vi "Convert PID Gains (PD).vi"(0 "proportional":sgl, 1 "gains pattern (Parallel)":T4=1 items=["Academic", "Parallel", "Series"], 2 "filter coefficient (NaN)":sgl=nan, 3 "filter coefficient unit (Alpha)":T1 items=["Alpha", "N", "Cutoff Frequency", "Time Constant"], 7 "derivative":sgl, 9 "sampling time":sgl min=0, 11 "error in (no error)":errorcluster, 12 "proportional unit (Gain (K))":T3 items=["Gain (K)", "Band (PB)"], 14 "derivative unit (s)":T2=1 items=["Hz", "s", "min"]) -> (4 "gains":T5 {"proportional gain" step=0.125}, 15 "error out":errorcluster)   [LabVIEW 2020]
doc: "Converts PID gains in the Academic, Parallel, or Series form to the normalized Parallel form that the PID VI expects."
uses:
  <vilib>/rvi/Analysis/control/PID/Typedef/niFpgaPID_PDGains.ctl
  <vilib>/rvi/Analysis/host/Private/PID Gains Pattern.ctl
  <vilib>/rvi/Analysis/host/Private/PID Proportional Unit.ctl
  <vilib>/rvi/Analysis/host/Private/PID Integral Derivative Unit.ctl
  <vilib>/rvi/Analysis/host/Private/PID Filter Coefficient Unit.ctl
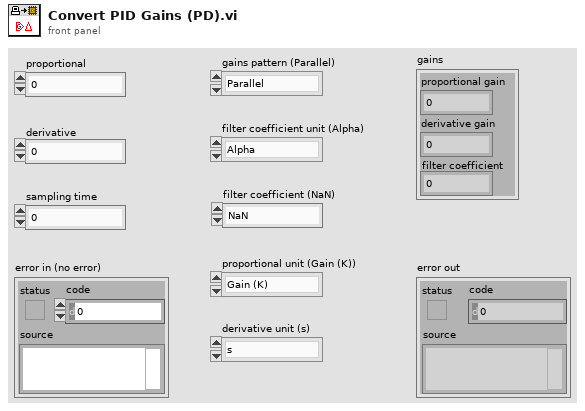
[diagram p1: front panel]
types:
  T1 = typedef "PID Filter Coefficient Unit.ctl" = u8
  T2 = typedef "PID Integral Derivative Unit.ctl" = u8
  T3 = typedef "PID Proportional Unit.ctl" = u8
  T4 = typedef "PID Gains Pattern.ctl" = u8
  T5 = typedef "niFpgaPID_PDGains.ctl" = cluster{"proportional gain":sgl, "derivative gain":sgl, "filter coefficient":sgl}
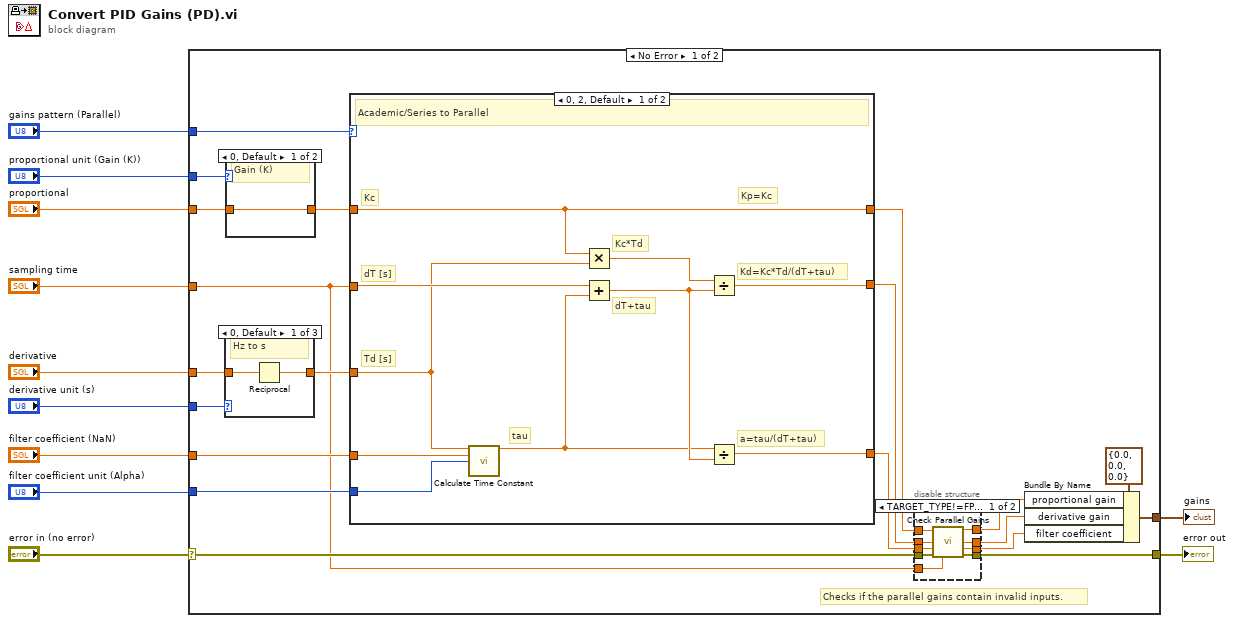
[diagram p0: block diagram]
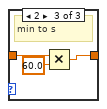
[diagram p4: hidden frame]
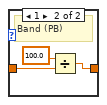
[diagram p5: hidden frame]
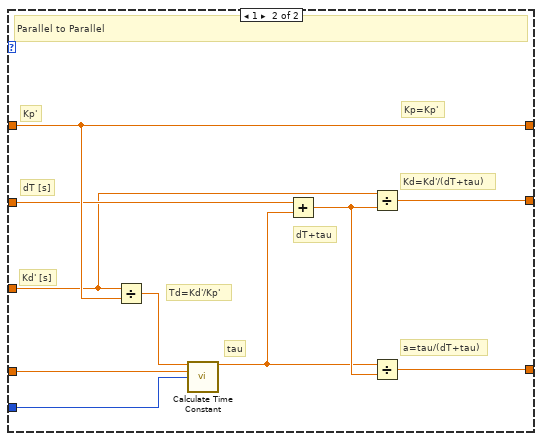
[diagram p6: hidden frame]
diagram:
  n1 = case shown="No Error" "error in (no error)" {
    selector: "error in (no error)" -> [w27 w75]
    tunnel: "gains pattern (Parallel)" -> [w31 _]
    tunnel: "filter coefficient (NaN)" -> [w30 _]
    tunnel: "sampling time" -> [w12 _]
    tunnel: "filter coefficient unit (Alpha)" -> [w29 _]
    tunnel: [w28 w75] -> w8
    tunnel: [w20 _] -> w7
    tunnel: "proportional" -> [w18 _]
    tunnel: "proportional unit (Gain (K))" -> [w17 _]
    tunnel: "derivative" -> [w14 _]
    tunnel: "derivative unit (s)" -> [w13 _]
    frame No Error {
      # "Checks if the parallel gains contain invalid inputs."
      n2 = case shown="0, Default" w13 {
        tunnel: w14 -> [w46 w47 w48]
        tunnel: [w45 w47 w49] -> w15
        frame 0, Default {
          # "Hz to s"
          n3 = Reciprocal(x=w46) -> (1/x=w45:sgl)
        }
        frame 1 {
          # "s to s"
        }
        frame 2 {
          # "min to s"
          n4 = Multiply(x=w48, y=sgl 60.0) -> (x*y=w49:sgl)
        }
      }
      n5 = case shown="0, Default" w17 {
        tunnel: w18 -> [w51 w52]
        tunnel: [w51 w54] -> w19
        frame 0, Default {
          # "Gain (K)"
        }
        frame 1 {
          # "Band (PB)"
          n6 = Divide(x=sgl 100.0, y=w52) -> (x/y=w54:sgl)
        }
      }
      n7 = case shown="0, 2, Default" w31 {
        tunnel: w19 -> [w59 w73]
        tunnel: w15 -> [w56 w69]
        tunnel: w30 -> [w57 w67]
        tunnel: w12 -> [w63 w72]
        tunnel: w29 -> [w58 w66]
        tunnel: [w64 w74] -> w24
        tunnel: [w59 w73] -> w26
        tunnel: [w60 w71] -> w25
        frame 0, 2, Default {
          # "Kp=Kc"
          # "Kd=Kc*Td/(dT+tau)"
          # "Kc*Td"
          # "dT+tau"
          # "a=tau/(dT+tau)"
          # "dT [s]"
          # "tau"
          # "Kc"
          # "Td [s]"
          # "Academic/Series to Parallel"
          n8 = call <vilib>:"Calculate Time Constant.vi"("derivative time"=w56, "filter coefficient (NaN)"=w57, "filter coefficient unit (Alpha)"=w58) -> ("time constant"=w55:sgl)  [unwired: 12 in]
          n9 = Multiply(x=w59, y=w56) -> (x*y=w62:sgl)
          n10 = Add(x=w63, y=w55) -> (x+y=w61:sgl)
          n11 = Divide(x=w62, y=w61) -> (x/y=w60:sgl)
          n12 = Divide(x=w55, y=w61) -> (x/y=w64:sgl)
        }
        frame 1 {
          # "Kp=Kp'"
          # "dT [s]"
          # "Kd=Kd'/(dT+tau)"
          # "dT+tau"
          # "tau"
          # "a=tau/(dT+tau)"
          # "Td=Kd'/Kp'"
          # "Kp'"
          # "Kd' [s]"
          # "Parallel to Parallel"
          n13 = Divide(x=w69, y=w73) -> (x/y=w68:sgl)
          n14 = call <vilib>:"Calculate Time Constant.vi"("derivative time"=w68, "filter coefficient (NaN)"=w67, "filter coefficient unit (Alpha)"=w66) -> ("time constant"=w65:sgl)  [unwired: 12 in]
          n15 = Add(x=w72, y=w65) -> (x+y=w70:sgl)
          n16 = Divide(x=w69, y=w70) -> (x/y=w71:sgl)
          n17 = Divide(x=w65, y=w70) -> (x/y=w74:sgl)
        }
      }
      n18 = disable-structure shown="TARGET_TYPE!=FPGA, Default" {
        disable-tunnel: [w40 w44] -> w28
        disable-tunnel: w27 -> [w39 w44]
        disable-tunnel: w26 -> [w38 w43]
        disable-tunnel: w25 -> [w37 w42]
        disable-tunnel: w24 -> [w36 w41]
        disable-tunnel: [w35 w41] -> w22
        disable-tunnel: [w34 w43] -> w21
        disable-tunnel: [w33 w42] -> w16
        disable-tunnel: w12 -> [w32 _]
        frame condition #0 (active) {
          n19 = call <vilib>:"Check Parallel Gains.vi"("proportional gain in"=w38, "derivative gain in (0)"=w37, "filter coefficient in (0)"=w36, "error in (no error)"=w39, "sampling time"=w32) -> ("proportional gain out"=w34:sgl, "derivative gain out"=w33:sgl, "filter coefficient out"=w35:sgl, "error out"=w40:errorcluster)  [unwired: 6 in, 1 out]
        }
        frame condition #1 {
        }
      }
      n20 = Bundle By Name(cluster=T5 {"proportional gain"=0.0, "derivative gain"=0.0, "filter coefficient"=0.0} ("gains"), "proportional gain"=w21, "derivative gain"=w16, "filter coefficient"=w22) -> (w20:T5)
    }
    frame Error {
    }
  }
  "error out" <- w8
  "gains" <- w7
